vi "Global Stop.vi"() -> ()   [LabVIEW 2018]
panel:
  out "Global Stop":bool
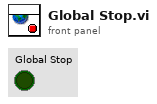
[diagram p1: front panel]
diagram:
